vi "ESP8266_DS18B20_Serial_LabVIEW.vi"() -> ()   [LabVIEW 2018]
doc: "This VI will continuously monitor the serial port and extract the temperature reading from the received string. This is stored in an array and displayed on the Graph. Press STOP to close the serial port and end the program.\n\nThis program is designed to work with the May 2009 version of the Arduino Temperature program which sends a header, the raw A/D value and the temperature as a float text value.\n\nSelect the appropriate COM port before running this VI. Leave the other serial port settings at their default values (9600, 8, none, 1.0, none)."
uses:
  <vilib>/Instr/_visa.llb/VISA Configure Serial Port (Instr).vi
panel:
  out "Temp2Array":dbl[](array[numeric]) caption="Temperature Array2"
  out "Temperature Graph 2":dbl[](graph)
  out "CurTemp2":dbl caption="Current Temperature2"
  out "concatenated string":string
  out "CurTemp1":dbl caption="Current Temperature1"
  in  "VISA resource name":refnum<visa-resource-name>="COM3"
  in  "baud rate (115200)":u32=115200
  in  "data bits (8)":u16=8 min=5 max=8 step=1
  in  "stop bits (10: 1 bit)":u16(ring)=10 items=["1.0"=10, "1.5"=15, "2.0"=20]
  in  "flow control (0:none)":u16(ring) items=["None", "XON/XOFF", "RTS/CTS", "XON/XOFF & RTS/CTS", "DTR/DSR", "XON/XOFF & DTR/DSR"]
  in  "parity (0:none)":enum16{"None", "Odd", "Even", "Mark", "Space"}(ring)
  in  "stop":bool
  out "Temp1Array":dbl[](array[numeric]) caption="Temperature Array1"
  out "Temperature Graph 1":dbl[](graph)
  # "This VI will continuously monitor the serial port and extract the temperature reading from the received string.  This is stored in an array and displayed on the Graph.  Press STOP to close the serial port and end the program.\n\nSelect the appropriate COM port before running this VI.  Leave the other serial port settings at their default values (115200, 8, none, 1.0, none)."
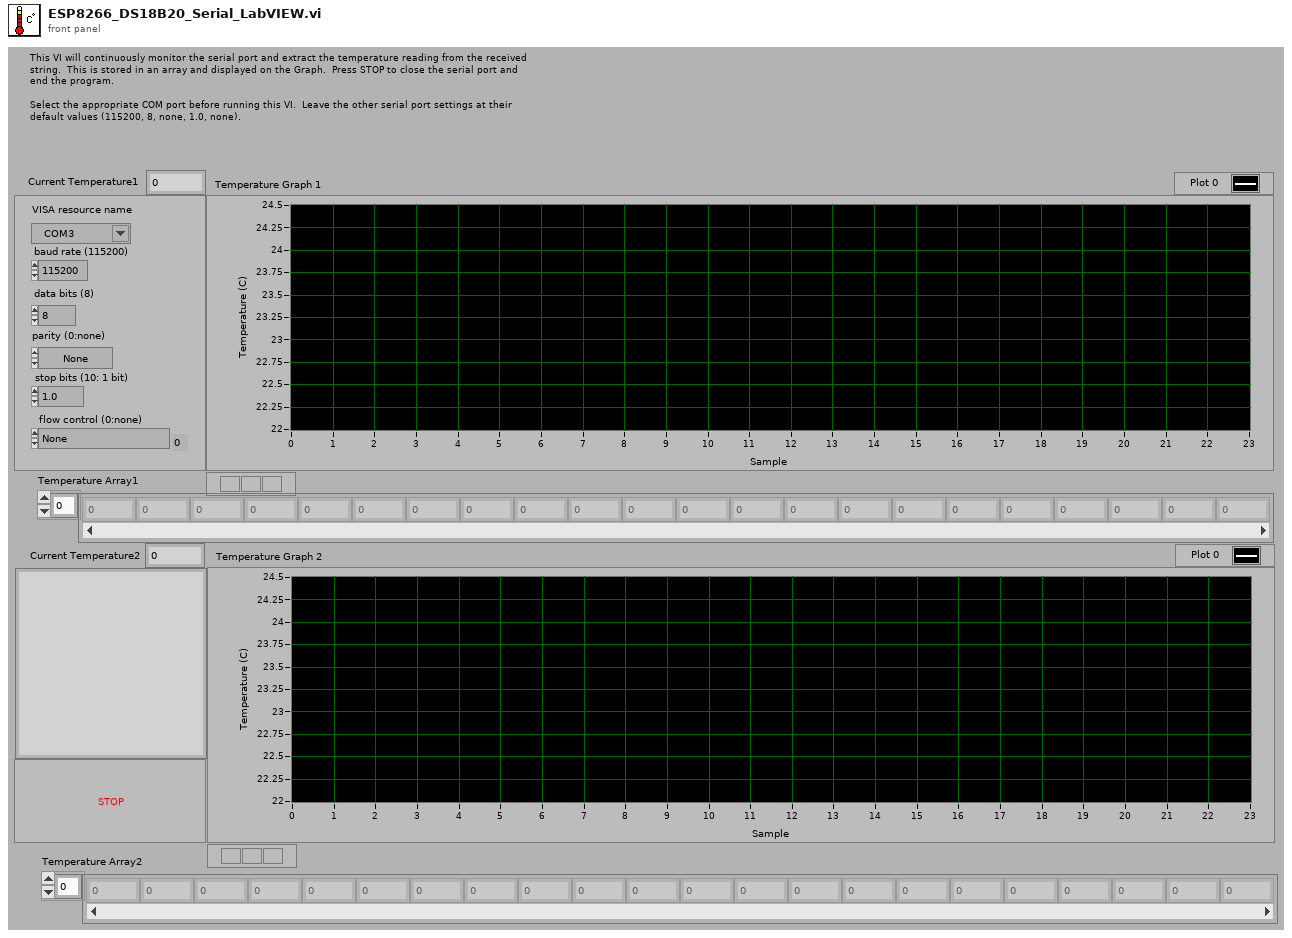
[diagram p1: front panel]
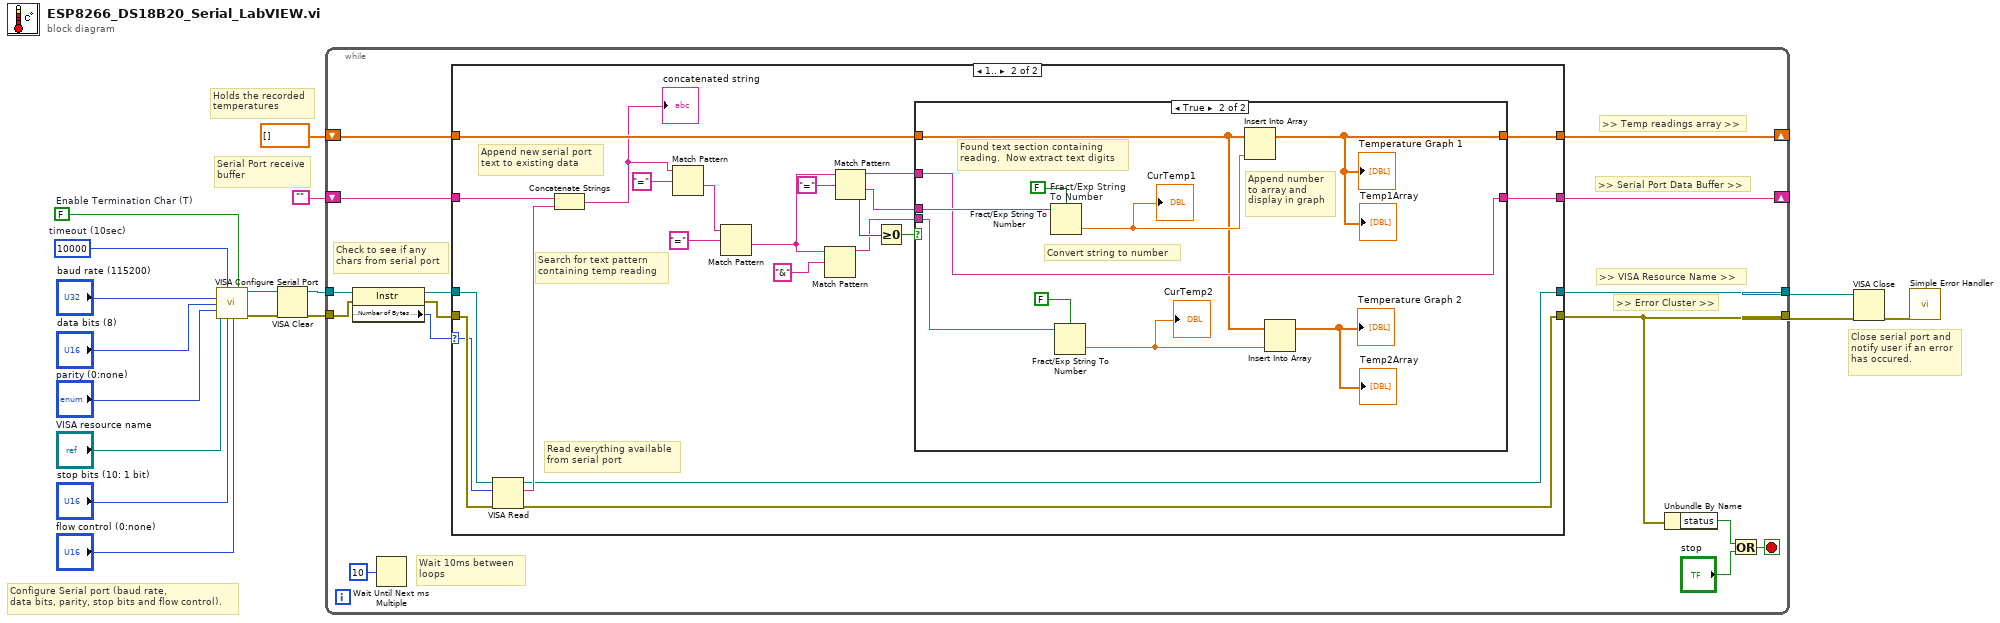
[diagram p0: block diagram]
diagram:
  w13 = FALSE  # Enable Termination Char (T)
  w14 = u32 10000  # timeout (10sec)
  # "Close serial port and\nnotify user if an error\nhas occured."
  # "Serial Port receive\nbuffer"
  # "Holds the recorded\ntemperatures"
  # "Configure Serial port (baud rate,\ndata bits, parity, stop bits and flow control)."
  n1 = call-poly "VISA Configure Serial Port"("VISA resource name"="VISA resource name", "timeout (10sec)"=w14, "Enable Termination\nChar (T)"=w13, "baud rate"="baud rate (115200)", "data bits (8)"="data bits (8)", "parity (0:none)"="parity (0:none)", "stop bits (10: 1 bit)"="stop bits (10: 1 bit)", "flow control (0:none)"="flow control (0:none)") -> ("VISA resource name out"=w11:refnum<visa-resource-name>, "error out"=w12:errorcluster)  [unwired: 6 in]
  n2 = VISA Clear(VISA resource name=w11, error in (no error)=w12) -> (VISA resource name out=w9:refnum<visa-resource-name>, error out=w8:errorcluster)
  n3 = while {
    tunnel: [w24] -> w17
    tunnel: [w32] -> w16
    shift-right: [w18] -> _
    shift-left: "" -> [w26]
    tunnel: w9 -> [w29]
    tunnel: w8 -> [w28]
    shift-right: [w20] -> _
    shift-left: dbl[] [] -> [w19]
    stop <- w23 stop-if-true
    # "Wait 10ms between \nloops"
    # ">> Error Cluster >>"
    # ">> VISA Resource Name >>"
    # ">> Temp readings array >>"
    # ">> Serial Port Data Buffer >>"
    # "Check to see if any\nchars from serial port"
    n4 = property class="Instr"(reference=w29, error in=w28) -> (reference out=w31:refnum<visa-resource-name>, error out=w30:errorcluster, "Serial Settings:Number of Bytes at Serial Port"=w27:u32)
    n5 = Wait Until Next ms Multiple(millisecond multiple=u32 10) -> ()  [unwired: 1 out]
    n6 = case shown="1.." w27 {
      selector: w27 -> [_ w54]
      tunnel: [w35 w39] -> w24
      tunnel: [w36 w40] -> w32
      tunnel: w31 -> [w36 w58]
      tunnel: w30 -> [w35 w57]
      tunnel: w26 -> [w34 w56]
      tunnel: [w34 w52] -> w18
      tunnel: [w33 w50] -> w20
      tunnel: w19 -> [w33 w51]
      frame 0, Default {
        # "No data in from serial port - Nothing to do."
      }
      frame 1.. {
        # "Search for text pattern\ncontaining temp reading"
        # "Append new serial port\ntext to existing data"
        # "Read everything available\nfrom serial port"
        n7 = VISA Read(VISA resource name=w58, byte count=w54, error in (no error)=w57) -> (VISA resource name out=w40:refnum<visa-resource-name>, read buffer=w55:string, error out=w39:errorcluster)  [unwired: 1 out]
        n8 = Concatenate Strings "Concatenate Strings"(w56, w55) -> (w43:string)
        "concatenated string" <- w43
        n9 = Match Pattern(string=w43, regular expression="=") -> (after substring=w48:string)  [unwired: 1 in, 3 out]
        n10 = Match Pattern(string=w48, regular expression="=") -> (after substring=w49:string)  [unwired: 1 in, 3 out]
        n11 = Match Pattern(string=w49, regular expression="&") -> (before substring=w38:string)  [unwired: 1 in, 3 out]
        n12 = Match Pattern(string=w49, regular expression="=") -> (before substring=w37:string, after substring=w42:string, offset past match=w41:i32)  [unwired: 1 in, 1 out]
        n13 = Greater Or Equal To 0?(x=w41) -> (x >= 0?=w53:bool)
        n14 = case shown="True" w53 {
          tunnel: w42 -> [w59 w68]
          tunnel: [w59 w65] -> w52
          tunnel: [w60 w70] -> w50
          tunnel: w51 -> [w60 w64]
          tunnel: w38 -> [_ w66]
          tunnel: w37 -> [_ w65]
          frame False {
            # "Did not find text pattern in the buffer.  Try again in the next loop after new data \nhas been received."
          }
          frame True {
            # "Append number\nto array and\ndisplay in graph"
            # "Convert string to number"
            # "Found text section containing \nreading.  Now extract text digits"
            n15 = Fract/Exp String To Number "Fract/Exp String \nTo Number"(use system decimal point (T)=FALSE, string=w68) -> (number=w69:dbl)  [unwired: 2 in, 1 out]
            "CurTemp1" <- w69
            n16 = Fract/Exp String To Number(use system decimal point (T)=FALSE, string=w66) -> (number=w63:dbl)  [unwired: 2 in, 1 out]
            "CurTemp2" <- w63
            n17 = Insert Into Array "Insert Into Array"(array=w64, new element=w69) -> (w70:dbl[])  [unwired: 1 in]
            "Temperature Graph 1" <- w70
            "Temp1Array" <- w70
            n18 = Insert Into Array "Insert Into Array"(array=w64, new element=w63) -> (→"Temperature Graph 2" →"Temp2Array":dbl[])  [unwired: 1 in]
          }
        }
      }
    }
    n19 = Unbundle By Name(w24) -> ("status"=w22:bool)
    n20 = Or(x=w22, y="stop") -> (x .or. y?=w23:bool)
  }
  n21 = VISA Close(VISA resource name=w16, error in (no error)=w17) -> (error out=w15:errorcluster)
  n22 = call <vilib>:"Simple Error Handler.vi"("error in (no error)"=w15) -> ()  [unwired: 4 in, 5 out]
